vi "Sample Main VI 1.vi"(11 "Radius":dbl) -> (3 "Circle Area":dbl)   [LabVIEW 2023]
doc: "This VI is used to demonstrate the addition of a VI to a project."
panel:
  # "Sample Main VI 1"
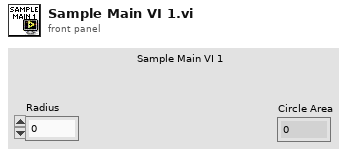
[diagram p1: front panel]
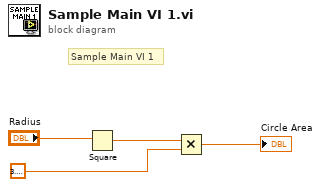
[diagram p0: block diagram]
diagram:
  # "Sample Main VI 1"
  n1 = Square(x="Radius") -> (x^2=w4:dbl)
  n2 = Multiply(x=w4, y=3.141592653589793) -> (x*y=→"Circle Area":dbl)
